vi "oax_gsBode Plot.vi"() -> ()   [LabVIEW 2017]
doc: "This is Order Analysis Toolkit demo VI."
uses:
  <vilib>/addons/Sound and Vibration/Order Analysis/Utility/SubVIs/oa_Buffer Settings.ctl
  <vilib>/addons/_NISVFA/_Spectrum Processing/SVFA Unit Conversion (XY) (N Ch).vi
  <vilib>/addons/Sound and Vibration/Order Analysis/Utility/OAT Output Buffered Data (XY, N Chan).vi
  <vilib>/addons/Sound and Vibration/Order Analysis/Resample Order Tracking/OAT Order Magnitude and Phase (Even Angle Signal, 1 Channel).vi
  <vilib>/addons/Sound and Vibration/Order Analysis/Resample Order Tracking/OAT Convert to Even Angle Signal (1 Channel).vi
  <vilib>/addons/Sound and Vibration/Order Analysis/Tach Process/OAT Analog Tacho Process (1 Tacho).vi
  <vilib>/Waveform/WDTOps.llb/WDT Waveform Duration DBL.vi
  <vilib>/addons/Sound and Vibration/Order Analysis/Utility/SoundVib_OAUtility.lvlib
  <vilib>/addons/Sound and Vibration/Order Analysis/Tach Process/SoundVib_TachProcess.lvlib
  <vilib>/addons/Sound and Vibration/Order Analysis/Resample Order Tracking/SoundVib_OrderTracking.lvlib
panel:
  in  "magnitude view":enum16{"no change", "rms", "peak", "peak-peak"}(ring)=enum."peak"
  in  "bandwidth [order]":dbl=1.0 format="%.2f"
  in  "buffer settings":T1={"buffer size"=10.0, "buffer unit"=enum."s"}
  in  "view":T2={"dB on? (F)"=FALSE, "unwrap phase? (T)"=TRUE, "unit in degree? (T)"=TRUE}
  in  "X axis selection":u16(ring) items=["Time", "Revolution", "RPM"]
  in  "orders to compute (1.0)":dbl[](array[numeric])=[1.0] format="%.2f"
  out "magnitude":T3(graph)
  out "phase":cluster{"X":dbl[], "Y":dbl[]}[](graph)
  in  "Select Data":i32(listbox)
  in  "STOP":bool
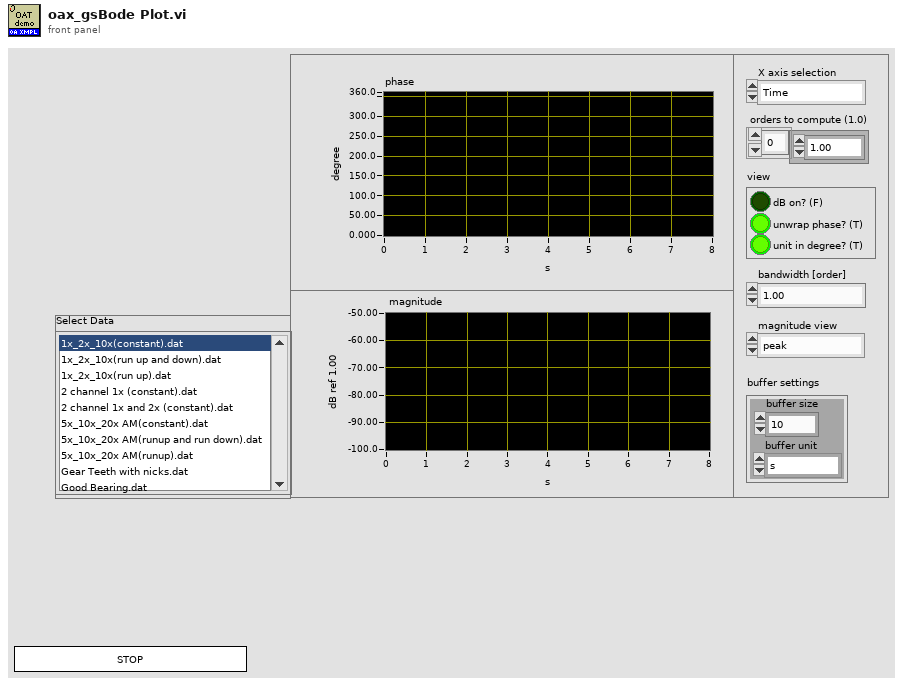
[diagram p1: front panel]
types:
  T1 = typedef "SoundVib_OAUtility.lvlib/oa_Buffer Settings.ctl" = cluster{"buffer size":dbl, "buffer unit":enum16{"s", "revolution", "# of samples"}}
  T2 = cluster{"dB on? (F)":bool, "unwrap phase? (T)":bool, "unit in degree? (T)":bool}
  T3 = cluster{"time/rev/rpm":dbl[], "magnitude":dbl[]}[]
  T4 = cluster{"linear/dB":enum16{"no change", "linear", "dB"}, "dB reference (0: no change)":dbl, "power/magnitude":enum16{"no change", "power", "magnitude"}, "view":enum16{"no change", "rms", "peak", "peak-peak"}}
  T5 = typedef "SoundVib_TachProcess.lvlib/speed profile.ctl" = cluster{"time [s]":dbl[], "speed [RPM]":dbl[]}
  T6 = typedef "OAT Position Info.ctl" = cluster{"positions [s]":dbl[], "samples/rev":dbl}
  T7 = typedef "svc_Resampled Channel Info.ctl" = cluster{"channel name":string, "description":string, " channel info":T8}
  T8 = typedef "svc_Channel Info.ctl" = cluster{"sensor sensitivity":dbl, "engineering units":T9, "dB reference":dbl, "custom label":string, "weighting filter":T10, "pregain":dbl}
  T9 = typedef "svc_Engineering Units Text Ring.ctl" = u16
  T10 = typedef "svc_Weighting Filter Text Ring.ctl" = u16
  T11 = cluster{"x unit":string, "magnitude unit":string, "phase unit":string}
  T12 = typedef "svc_Spectrum Info.ctl" = cluster{"channel name":string, "description":string, "x-axis units":T13, "spectral info":cluster{"spectrum type":T14, "linear/dB":enum16{"linear", "dB"}, "window":u16, "window size":i32, "FFT size":i32}, "engineering units":T9, "custom label":string, "dB reference [EU]":dbl, "peak units":enum16{"rms", "peak", "peak-peak"}, "weighting filter":T10, "spectral density?":bool, "unit label":string, "spectrum skewed?":bool, "complimentary spectrum units":T15}
  T13 = typedef "svc_X-Axis Units.ctl" = u16
  T14 = typedef "svc_Spectrum Type.ctl" = enum16{"FFT Spectrum [complex]", "Amplitude [Magnitude]", "Power [Magnitude^2]", "Cross Spectrum [complex]", "Frequency Response [Complex]"}
  T15 = typedef "svc_Complimentary Spectrum Units.ctl" = enum16{"none", "radians", "degrees", "cycles", "imaginary"}
  T16 = cluster{"pulse / rev":i32, "threshold (auto)":dbl, "slope (Rising)":u16}
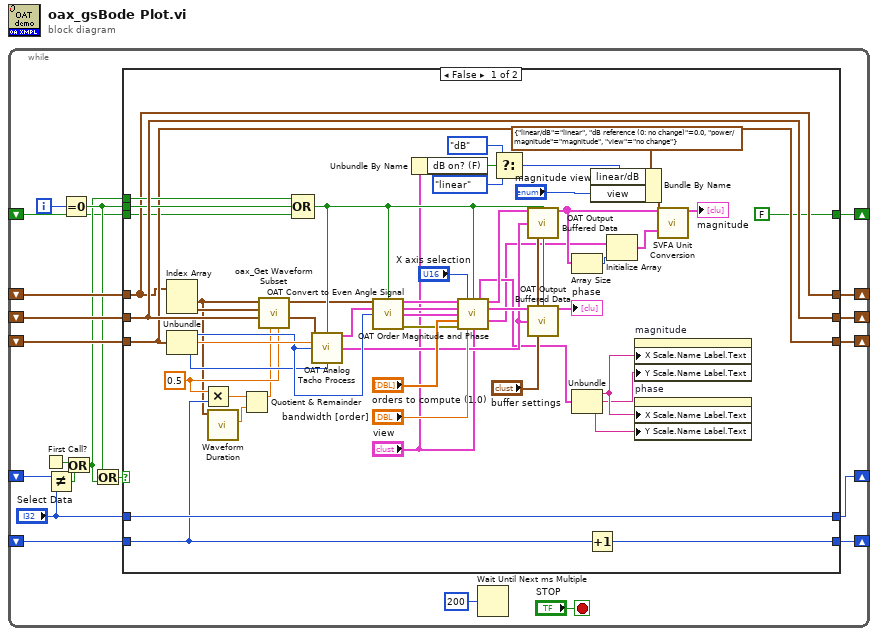
[diagram p0: block diagram]
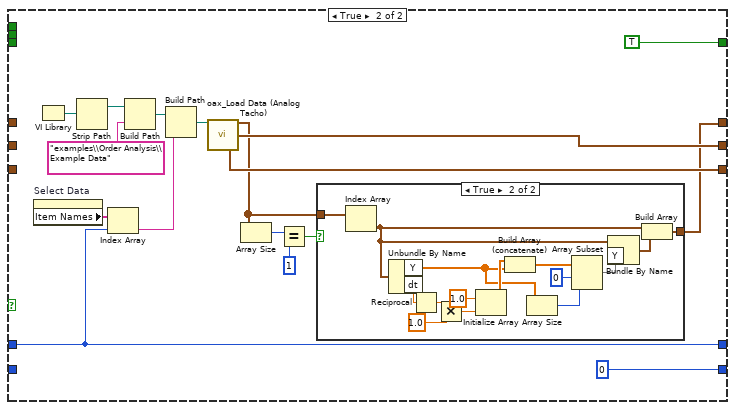
[diagram p2: hidden frame]
diagram:
  n1 = while {
    shift-right: [w17] -> _
    shift-left: _ -> [w18]
    shift-right: [w15] -> _
    shift-left: _ -> [w21]
    shift-right: [w14] -> _
    shift-left: _ -> [w19]
    shift-right: [w13] -> _
    shift-left: _ -> [w12]
    shift-right: [w3] -> _
    shift-left: _ -> [w4]
    shift-right: [w2] -> _
    shift-left: _ -> [w1]
    i -> [w11]
    stop <- "STOP" stop-if-true
    n2 = First Call?() -> (First Call?: T/F=w7:bool)
    n3 = Not Equal?(x=w18, y="Select Data") -> (x != y?=w6:bool)
    n4 = Equal To 0?(x=w11) -> (x = 0?=w10:bool)
    n5 = Or(x=w7, y=w6) -> (x .or. y?=w5:bool)
    n6 = Or(x=w10, y=w5) -> (x .or. y?=w9:bool)
    n7 = case shown="False" w9 {
      tunnel: w21 -> [w53 _]
      tunnel: w19 -> [w71 _]
      tunnel: [w72 w89] -> w17
      tunnel: "Select Data" -> [w72 w89]
      tunnel: [w53 w74] -> w15
      tunnel: [w71 w87] -> w14
      tunnel: [w64 w86] -> w13
      tunnel: w12 -> [w64 _]
      tunnel: w5 -> [w69 _]
      tunnel: w10 -> [w68 _]
      tunnel: w4 -> [w58 _]
      tunnel: [w60 0] -> w3
      tunnel: [FALSE TRUE] -> w2
      tunnel: w1 -> [w52 _]
      frame False {
        w59 = 0.5 ("y")
        n8 = Index Array(array=w53) -> (element #1=w57:waveform(dbl), element #2=w65:waveform(dbl))  [unwired: 2 in]
        n9 = Unbundle(w64) -> ("pulse / rev"=w62:i32, "threshold (auto)"=w63:dbl, "slope (Rising)"=w61:u16)
        n10 = Multiply(x=w59, y=w58) -> (x*y=w55:dbl)
        n11 = call-poly <vilib>:"Waveform Duration.vi"("waveform in"=w57) -> ("duration"=w56:dbl)  [unwired: 8 in, 2 out]
        n12 = Quotient & Remainder(x=w55, y=w56) -> (x-y*floor(x/y)=w54:dbl)  [unwired: 1 out]
        n13 = call <vilib>:"oax_Get Waveform Subset.vi"("duration"=w59, "start index"=w54, "Tach Signal"=w71, "Vibration Signal Y"=w65, "Vibration Signal X"=w57) -> ("Tach Signal out"=w70:waveform(dbl), "Vibration Signal X out"=w66:waveform(dbl))  [unwired: 3 in, 2 out]
        n14 = Compound Arithmetic op=OR(w69, w68, w52) -> (w67:bool)
        n15 = call-poly <vilib>:"OAT Analog Tacho Process.vi"("analog tacho signal"=w70, "reset? (F)"=w67, "threshold (auto)"=w63, "pulse/revolution (1)"=w62, "slope (Rising)"=w61) -> ("speed profile"=w73:T5, "speed position info"=w32:T6)  [unwired: 6 in, 3 out]
        n16 = call-poly <vilib>:"OAT Convert to Even Angle Signal.vi"("scaled signal [EU]"=w66, "reset? (F)"=w67, "speed profile"=w73, "pulse/revolution (1)"=w62) -> ("even-angle signal"=w48:cluster{"r0":dbl, "dr":dbl, "Y":dbl[]}, "even-angle channel info"=w47:T7, "even-angle position info"=w41:T6, "error out"=w46:errorcluster)  [unwired: 7 in, 1 out]
        n17 = Unbundle By Name("view") -> ("dB on? (F)"=w26:bool)
        n18 = call-poly <vilib>:"OAT Order Magnitude and Phase.vi"("even-angle signal"=w48, "x-axis selection"="X axis selection", "reset? (F)"=w67, "even-angle channel info"=w47, "even-angle position info"=w41, "orders to compute (1.0)"="orders to compute (1.0)", "error in (no error)"=w46, "bandwidth [order]"="bandwidth [order]", "view"="view") -> ("unit labels"=w31:T11, "magnitudes [RMS]"=w43:T3, "phases [phase lag]"=w45:cluster{"time/rev/rpm":dbl[], "phase":dbl[]}[], "magnitude info"=w22:T12)  [unwired: 1 in, 2 out]
        n19 = Select(t=enum16{"no change", "linear", "dB"}."dB" ("linear/dB"), s=w26, f=enum16{"no change", "linear", "dB"}."linear" ("linear/dB")) -> (s? t:f=w23:enum16{"no change", "linear", "dB"})
        n20 = call-poly <vilib>:"OAT Output Buffered Data.vi"("XY signals"=w43, "reset? (F)"=w67, "position info"=w32, "buffer settings"="buffer settings") -> ("buffered XY signals"=w38:cluster{"X":dbl[], "Y":dbl[]}[])  [unwired: 9 in, 2 out]
        n21 = call-poly <vilib>:"OAT Output Buffered Data.vi"("XY signals"=w45, "reset? (F)"=w67, "position info"=w32, "buffer settings"="buffer settings") -> ("buffered XY signals"=→"phase":cluster{"X":dbl[], "Y":dbl[]}[])  [unwired: 9 in, 2 out]
        n22 = Array Size(array=w38) -> (size(s)=w37:i32)
        n23 = Unbundle(w31) -> ("x unit"=w30:string, "magnitude unit"=w29:string, "phase unit"=w28:string)
        n24 = Increment(x=w58) -> (x+1=w60:i32)
        n25 = Bundle By Name(cluster=T4 {"linear/dB"=enum."linear", "dB reference (0: no change)"=0.0, "power/magnitude"=enum."magnitude", "view"=enum."no change"} ("desired scaling"), "linear/dB"=w23, "view"="magnitude view") -> (w34:T4)
        n26 = Initialize Array(w22, w37) -> (w36:T12[])
        n27 = property on="magnitude" class="XYGraph (strict)"("X Scale.Name Label.Text"=w30, "Y Scale.Name Label.Text"=w29) -> ()  [unwired: 2 in, 2 out]
        n28 = property on="phase" class="XYGraph (strict)"("X Scale.Name Label.Text"=w30, "Y Scale.Name Label.Text"=w28) -> ()  [unwired: 2 in, 2 out]
        n29 = call-poly <vilib>:"SVFA Unit Conversion.vi"("magnitudes"=w38, "desired scaling"=w34, "magnitudes info in"=w36) -> ("converted magnitudes"=→"magnitude":T3)  [unwired: 13 in, 3 out]
      }
      frame True {
        n30 = property on="Select Data" class="LstBox (strict)"() -> ("Item Names"=w90:string[])  [unwired: 2 in, 2 out]
        n31 = VI Library() -> (path=w82:path)
        n32 = Strip Path(path=w82) -> (stripped path=w81:path)  [unwired: 1 out]
        n33 = Index Array(array=w90, index=w89) -> (element=w84:string)
        n34 = Build Path(base path=w81, name or relative path="examples\\Order Analysis\\Example Data") -> (appended path=w85:path)
        n35 = Build Path(base path=w85, name or relative path=w84) -> (appended path=w83:path)
        n36 = call <vilib>:"oax_Load Data (Analog Tacho).vi"("Data Path In"=w83) -> ("vibration data"=w75:waveform(dbl)[], "analog tacho signal"=w87:waveform(dbl), "tacho info"=w86:T16)  [unwired: 8 in, 4 out]
        n37 = Array Size(array=w75) -> (size(s)=w78:i32)
        n38 = Equal?(x=w78, y=1) -> (x = y?=w76:bool)
        n39 = case shown="True" w76 {
          tunnel: w75 -> [w91 w106]
          tunnel: [w91 w105] -> w74
          frame False {
          }
          frame True {
            n40 = Index Array(array=w106) -> (element=w104:waveform(dbl))  [unwired: 1 in]
            n41 = Unbundle By Name(w104) -> ("Y"=w93:dbl[], "dt"=w102:dbl)
            n42 = Reciprocal(x=w102) -> (1/x=w101:dbl)
            n43 = Multiply(x=w101, y=1.0) -> (x*y=w99:dbl)
            n44 = Initialize Array(1.0 ("element"), w99) -> (w95:dbl[])
            n45 = Build Array (concatenate)(w95, w93) -> (w97:dbl[])
            n46 = Array Size(array=w93) -> (size(s)=w94:i32)
            n47 = Array Subset(array=w97, index=0, length=w94) -> (w92:dbl[])
            n48 = Bundle By Name(cluster=w104, "Y"=w92) -> (w103:waveform(dbl))
            n49 = Build Array(w104, w103) -> (w105:waveform(dbl)[])
          }
        }
      }
    }
    n50 = Wait Until Next ms Multiple(millisecond multiple=u32 200) -> ()  [unwired: 1 out]
  }
